vi "MSScript_SubVI_VarTypeIden.vi"(1 "Var in":string="@Array[$abc]") -> (0 "Type":T1(ring))   [LabVIEW 2018, in "MSScript.lvclass"]
uses:
  MSScript.lvclass
  <vilib>/regexp/Match Regular Expression.xnode
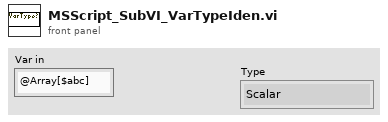
[diagram p1: front panel]
types:
  T1 = enum16{"Scalar", "ScalarArray", "Var", "VarArray", "Error"}
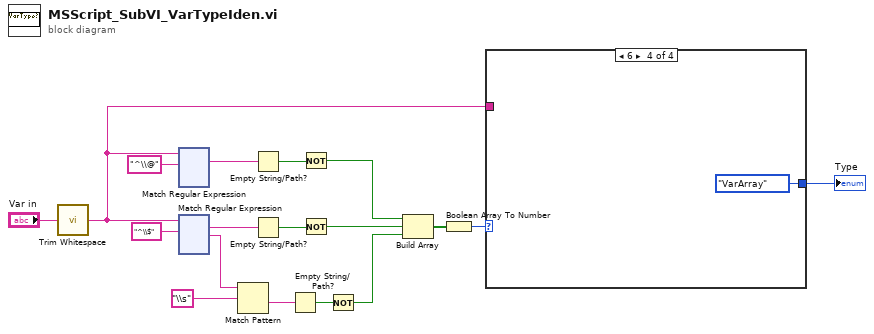
[diagram p0: block diagram]
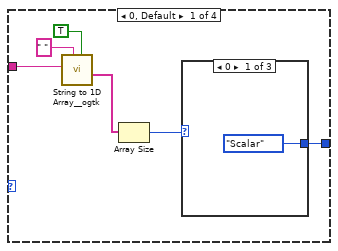
[diagram p2: hidden frame]
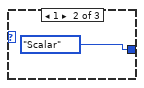
[diagram p3: hidden frame]
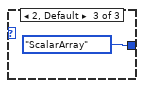
[diagram p4: hidden frame]
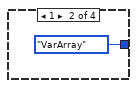
[diagram p5: hidden frame]
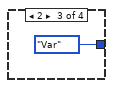
[diagram p6: hidden frame]
diagram:
  n1 = call <vilib>:"Trim Whitespace.vi"("string"="Var in") -> ("trimmed string"=w7:string)  [unwired: 1 in]
  n2 = xnode "Match Regular Expression"("input string"=w7, "regular expression"="^\\@") -> ("whole match"=w15:string)  [unwired: 4 in, 4 out]
  n3 = xnode "Match Regular Expression"("input string"=w7, "regular expression"="^\\$") -> ("whole match"=w14:string, "after match"=w5:string)  [unwired: 4 in, 3 out]
  n4 = Match Pattern(string=w5, regular expression="\\s") -> (after substring=w3:string)  [unwired: 1 in, 3 out]
  n5 = Empty String/Path?(string/path=w15) -> (empty?=w13:bool)
  n6 = Empty String/Path?(string/path=w14) -> (empty?=w12:bool)
  n7 = Empty String/Path?(string/path=w3) -> (empty?=w2:bool)
  n8 = Not(x=w13) -> (.not. x?=w11:bool)
  n9 = Not(x=w12) -> (.not. x?=w10:bool)
  n10 = Not(x=w2) -> (.not. x?=w1:bool)
  n11 = Build Array(w11, w10, w1) -> (w9:bool[])
  n12 = Boolean Array To Number(Boolean array=w9) -> (number=w8:u32)
  n13 = case shown="6" w8 {
    tunnel: [w19 T1."VarArray" T1."Var" T1."VarArray"] -> w6
    tunnel: w7 -> [w24 _ _ _]
    frame 0, Default {
      n14 = call <userlib>:"String to 1D Array__ogtk.vi"("ignore duplicate delimiters? (F=No)"=TRUE, "delimiter (Tab)"=" ", "string"=w24) -> ("Array of Strings"=w21:string[])  [unwired: 8 in]
      n15 = Array Size(array=w21) -> (size(s)=w20:i32)
      n16 = case shown="0" w20 {
        tunnel: [T1."Scalar" T1."Scalar" T1."ScalarArray"] -> w19
        frame 0 {
        }
        frame 1 {
        }
        frame 2, Default {
        }
      }
    }
    frame 1 {
    }
    frame 2 {
    }
    frame 6 {
    }
  }
  "Type" <- w6
